vi "Write Block.vi"(8 "Error In":errorcluster, 10 "Bytes":u8[](array[numeric]), 11 "SFTP File In":refnum<class "SFTP File.lvclass">) -> (0 "Error Out":errorcluster, 2 "Block Write Count":i64, 3 "SFTP File Out":refnum<class "SFTP File.lvclass">)   [LabVIEW 2018, in "Toolkit.lvlib" / "SFTP File.lvclass"]
uses:
  SFTP File.lvclass
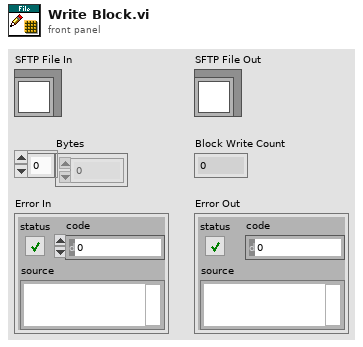
[diagram p1: front panel]
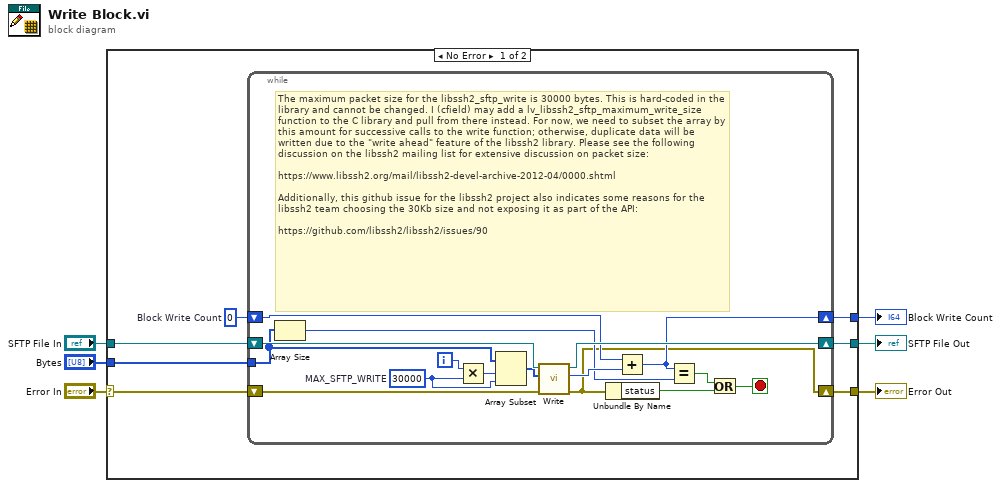
[diagram p0: block diagram]
diagram:
  n1 = case shown="No Error" "Error In" {
    selector: "Error In" -> [w7 w30]
    tunnel: "Bytes" -> [w12 _]
    tunnel: "SFTP File In" -> [w11 w31]
    tunnel: [w10 _] -> w4
    tunnel: [w9 w31] -> w3
    tunnel: [w8 w30] -> w2
    frame No Error {
      w13 = i64 0  # Block Write Count
      n2 = while {
        tunnel: w12 -> [w22]
        shift-right: [w27] -> w9
        shift-left: w11 -> [w29]
        shift-right: [w15] -> w8
        shift-left: w7 -> [w28]
        shift-right: [w24] -> w10
        shift-left: w13 -> [w26]
        i -> [w21]
        stop <- w16 stop-if-true
        w19 = 30000  # MAX_SFTP_WRITE
        # "The maximum packet size for the libssh2_sftp_write is 30000 bytes. This is hard-coded in the library and cannot be changed. I (cfield) may add a lv_libssh2_sftp_maximum_write_size function to the C library and pull from there instead. For now, we need to subset the array by this amount for successive calls to the write function; otherwise, duplicate data will be written due to the \"write ahead\" feature of the libssh2 library. Please see the following discussion on the libssh2 mailing list for extensive discussion on packet size:\n\nhttps://www.libssh2.org/mail/libssh2-devel-archive-2012-04/0000.shtml\n\nAdditionally, this github issue for the libssh2 project also indicates some reasons for the libssh2 team choosing the 30Kb size and not exposing it as part of the API:\n\nhttps://github.com/libssh2/libssh2/issues/90"
        n3 = Array Size(array=w22) -> (size(s)=w23:i32)
        n4 = Multiply(x=w21, y=w19) -> (x*y=w20:i32)
        n5 = Array Subset(array=w22, index=w20, length=w19) -> (w18:u8[])
        n6 = call "Write.vi"("Error In"=w28, "Data"=w18, "SFTP File In"=w29) -> ("Error Out"=w15:errorcluster, "Count"=w25:i64, "SFTP File Out"=w27:refnum<class "SFTP File.lvclass">)  [unwired: 6 in]
        n7 = Unbundle By Name(w15) -> ("status"=w14:bool)
        n8 = Add(x=w26, y=w25) -> (x+y=w24:i64)
        n9 = Equal?(x=w24, y=w23) -> (x = y?=w17:bool)
        n10 = Or(x=w17, y=w14) -> (x .or. y?=w16:bool)
      }
    }
    frame Error {
    }
  }
  "Block Write Count" <- w4
  "SFTP File Out" <- w3
  "Error Out" <- w2
